vi "Transform Enum.vi"(10 "String":string, 11 "Message":T1=enum."Load Data") -> (2 "Message out":T1=enum."Load Data", 3 "Message String":string)   [LabVIEW 2020, in "Main_Process.lvlib" / "Internal Messaging Library.lvlib"]
uses:
  Internal Messaging Library.lvlib
  Controls/Message.ctl
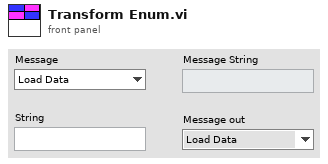
[diagram p1: front panel]
types:
  T1 = typedef "Main_Process.lvlib/Internal Messaging Library.lvlib/Message.ctl" = enum16{"Initialize", "Exit", "Error", "Load Data", "Add Time Entry", "Modify Time Entry", "Delete Time Entry"}
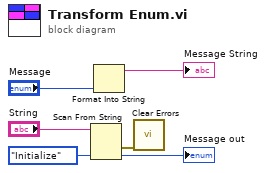
[diagram p0: block diagram]
diagram:
  n1 = Scan From String(input string="String", default 1=Message."Initialize" ("Message out")) -> (error out=w1:errorcluster, output 1=→"Message out":T1)  [unwired: 3 in, 2 out]
  n2 = Format Into String("Message") -> (resulting string=→"Message String":string)  [unwired: 3 in, 1 out]
  n3 = call <vilib>:"Clear Errors.vi"("error in (no error)"=w1) -> ()  [unwired: 5 in, 2 out]
